vi "Initialize Master.vi"(8 "error in (no error)":errorcluster, 11 "serial master in":refnum<class "Serial Master.lvclass">) -> (0 "error out":errorcluster, 3 "serial master out":refnum<class "Serial Master.lvclass">)   [LabVIEW 2018, in "SubVIs.lvlib" / "Serial Master.lvclass"]
doc: "This provides an interface for the master to open a connection to the slave."
uses:
  Serial Master.lvclass
  Serial Master.lvclass/Serial Master.ctl
  Transmission Data Unit.lvclass/Transmission Data Unit.ctl
  Read VISA resource name.vi
  Read Serial Data Unit.vi
  Read Baud Rate.vi
  Read Parity.vi
  Read Flow Control.vi
  Serial Data Unit.lvclass
  C:/OCC/ICM/Source Distributions/Buses/Transmission Data Unit.lvclass
  Serial Shared Components.lvlib
  Transmission Data Unit.lvclass
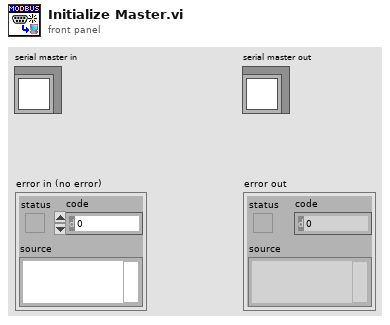
[diagram p1: front panel]
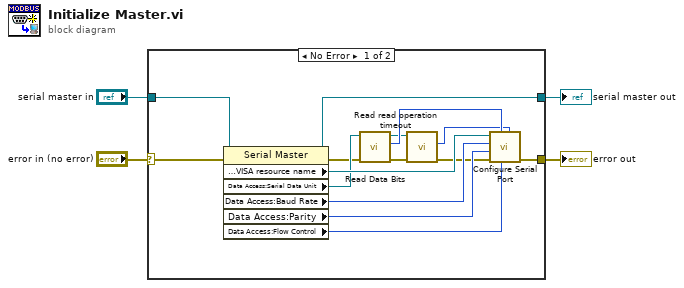
[diagram p0: block diagram]
diagram:
  n1 = case shown="No Error" "error in (no error)" {
    selector: "error in (no error)" -> [w8 w21]
    tunnel: "serial master in" -> [w19 w20]
    tunnel: [w14 w20] -> w3
    tunnel: [w13 w21] -> w2
    frame No Error {
      n2 = property class="Serial Master"(reference=w19, error in=w8) -> (reference out=w14:refnum<class "Serial Master.lvclass">, error out=w16:errorcluster, "Data Access:VISA resource name"=w18:refnum<visa-resource-name>, "Data Access:Serial Data Unit"=w17:refnum<class "Serial Data Unit.lvclass">, "Data Access:Baud Rate"=w11:u32, "Data Access:Parity"=w10:u16, "Data Access:Flow Control"=w9:u16)
      n3 = call-dynamic "Read Data Bits.vi"("error in (no error)"=w16, "serial data unit in"=w17) -> ("error out"=w15:errorcluster, "data bits"=w12:u16, "serial data unit out"=w6:refnum<class "Serial Data Unit.lvclass">)  [unwired: 7 in]
      n4 = call "Read read operation timeout.vi"("error in (no error)"=w15, "transmission data unit in"=w6) -> ("error out"=w7:errorcluster, "read operation timeout"=w5:i32)  [unwired: 7 in, 1 out]
      n5 = call "Configure Serial Port.vi"("Timeout"=w5, "flow control"=w9, "data bits"=w12, "error in (no error)"=w7, "parity"=w10, "baud rate"=w11, "VISA refnum in"=w18) -> ("error out"=w13:errorcluster)  [unwired: 4 in]
    }
    frame Error {
    }
  }
  "error out" <- w2
  "serial master out" <- w3
